vi "Read Thread States.vi"(8 "error in (no error)":errorcluster, 11 "Framework in":refnum<class "Framework.lvclass">) -> (0 "error out":errorcluster, 1 "private thread states":T1[](array[typedef]), 2 "public thread states":T1[](array[typedef]), 3 "Framework out":refnum<class "Framework.lvclass">)   [LabVIEW 2019, in "DSF Core.lvlib" / "Framework.lvclass"]
uses:
  Framework.lvclass
  Thread/Thread State.ctl
  Framework.lvclass/Framework.ctl
  Thread Manager/Thread Manager.lvclass/Thread Manager.ctl
  <vilib>/NI/Memory Manager/Classes/Pointer/Pointer.lvclass/Pointer.ctl
  <vilib>/NI/Memory Manager/Classes/Pointer/Read.vi
  <vilib>/NI/Memory Manager/Classes/Pointer/Read 1D U8.vi
  <vilib>/NI/Memory Manager/Classes/Pointer/Read (No Check).vi
  <vilib>/NI/Memory Manager/Classes/Pointer/Read (No Check) 1D U8.vi
  <vilib>/NI/Memory Manager/Classes/Pointer/Check Move.vi
  <vilib>/NI/Memory Manager/Classes/Pointer/Get Address.vi
  <vilib>/NI/Memory Manager/Classes/Pointer/Check Null Pointer.vi
  <vilib>/NI/Memory Manager/Classes/Pointer/Check Count.vi
  <vilib>/NI/Memory Manager/Classes/Pointer/Check Bounds (Power of 2).vi
  <vilib>/NI/Memory Manager/Classes/Pointer/Errors.vi
  <vilib>/NI/Memory Manager/Classes/Pointer/Null Pointer.vi
  <vilib>/NI/Memory Manager/Classes/Pointer/Is Null.vi
  <vilib>/NI/Memory Manager/Classes/Pointer/Get Size.vi
  <vilib>/NI/Memory Manager/Classes/Pointer/Out of Bounds.vi
  <vilib>/NI/Memory Manager/Classes/Pointer/Check Bounds.vi
  <vilib>/NI/Memory Manager/Classes/Pointer/Create Error.vi
  <vilib>/NI/Memory Manager/VIs/Write String to Source.vi
  <vilib>/NI/Memory Manager/Classes/Pointer/Write Pointer Size to Error.vi
  <vilib>/NI/Memory Manager/VIs/Write Numeric to Source.vi
  <vilib>/NI/Memory Manager/VIs/Write Numeric Scalar to Source (Base10 U64).vi
  <vilib>/NI/Memory Manager/Classes/Pointer/Check Bounds (Pointer).vi
  <vilib>/NI/Memory Manager/Classes/Pointer/Check Bounds (Buffer).vi
  <vilib>/NI/Memory Manager/VIs/New Error Cluster.vi
  <vilib>/NI/Memory Manager/VIs/New Error Cluster (512B).vi
  <vilib>/NI/Memory Manager/VIs/Set Error Status.vi
  <vilib>/NI/Memory Manager/VIs/Set Error Code.vi
  <vilib>/NI/Memory Manager/VIs/Set Error Source.vi
  <vilib>/NI/Memory Manager/Constants/Constants.vi
  <vilib>/NI/Memory Manager/Constants/Library Name.vi
  <vilib>/NI/Memory Manager/Classes/Pointer/Pointer Error Info.vi
  <vilib>/NI/Memory Manager/Constants/Pointer Class Name.vi
  <vilib>/NI/Memory Manager/Classes/Pointer/Buffer Underflow.vi
  Thread Manager/Thread Manager.lvclass
  Thread/Thread.lvclass
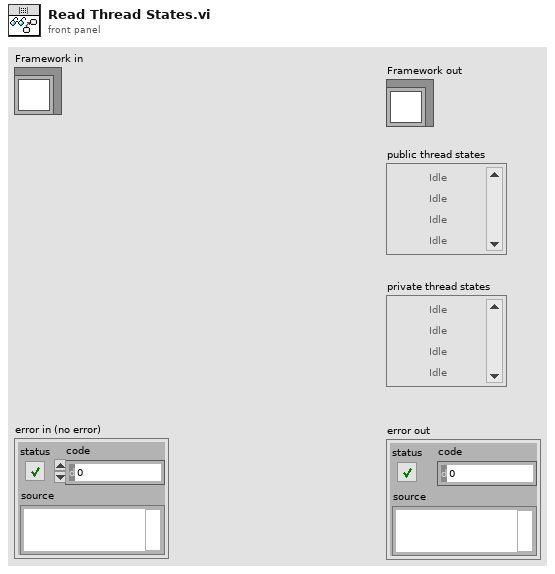
[diagram p1: front panel]
types:
  T1 = typedef "DSF Core.lvlib/Thread.lvclass/Thread State.ctl" = enum8{"Idle", "Running", "Error", "Shut Down"}
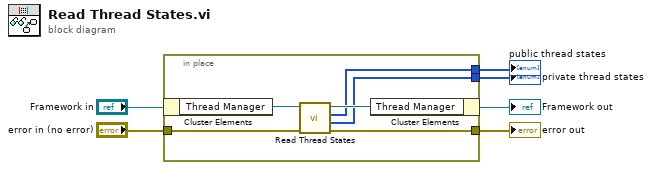
[diagram p0: block diagram]
diagram:
  n1 = in-place {
    in-place-border: "error in (no error)" -> [w10]
    in-place-border: [w9] -> w4
    in-place-border: [w8] -> w5
    in-place-border: [w7] -> w6
    n2 = in-place-cluster #1("Framework in") -> ("Thread Manager"=w12:refnum<class "Thread Manager.lvclass">)
    n3 = call "Read Thread States.vi"("error in (no error)"=w10, "Thread Manager in"=w12) -> ("error out"=w9:errorcluster, "private thread states"=w8:T1[], "public thread states"=w7:T1[], "Thread Manager out"=w11:refnum<class "Thread Manager.lvclass">)  [unwired: 6 in]
    n4 = in-place-cluster #1("Thread Manager"=w11) -> (→"Framework out":refnum<class "Framework.lvclass">)
  }
  "public thread states" <- w6
  "private thread states" <- w5
  "error out" <- w4
